vi "Post Build Script (G-CLI build).vi"(5 "create 7zip.bat only [T]":bool=TRUE, 6 "Package LabVIEW Version (19.0 (32-bit))":string, 7 "Project File Path":path, 8 "Package Source Folder":path, 9 "Package Version (major.minor.patch.build)":string, 10 "Product Name":string, 11 "Output Package File Path":path) -> (0 "error out":errorcluster)   [LabVIEW 2019, in "PostBuildSupport.lvclass"]
doc: "After you manually build the Application and Installer inside your project, you can then call this VI to create single self-extracting installer file. It is meant to be placed inside \"Post-Build Custom Action.vi\" that is called post VIPM package build."
uses:
  PostBuildSupport.lvclass
  PostBuildSupport.lvclass/PostBuildSupport.ctl
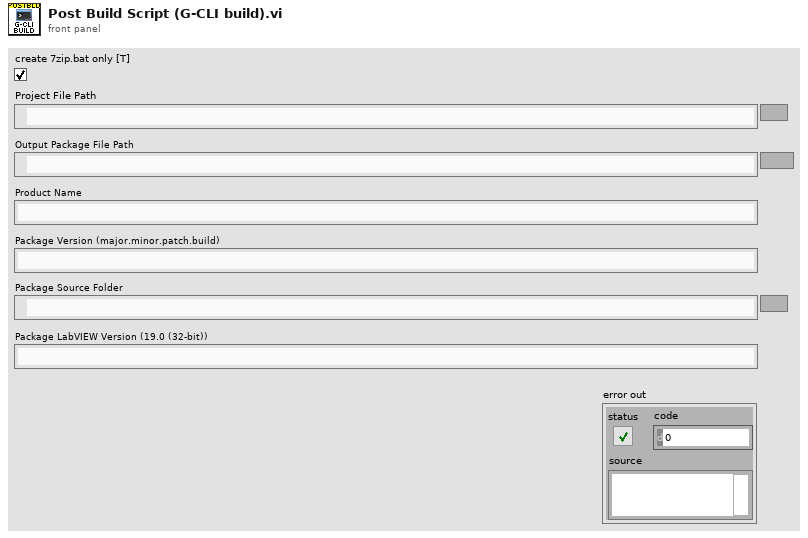
[diagram p1: front panel]
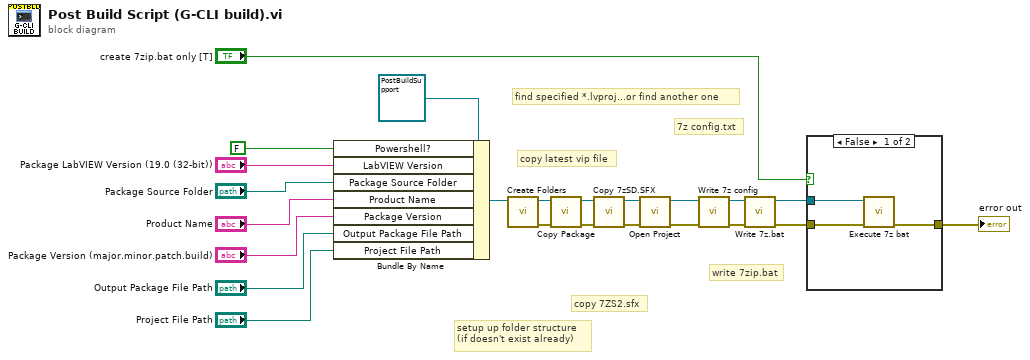
[diagram p0: block diagram]
diagram:
  # "find specified *.lvproj...or find another one"
  # "copy 7ZS2.sfx"
  # "setup up folder structure \n(if doesn't exist already)"
  # "copy latest vip file"
  # "7z config.txt"
  # "write 7zip.bat"
  n1 = Bundle By Name(cluster=refnum<class "PostBuildSupport.lvclass"> refnum ("PostBuildSupport in"), "Powershell?"=FALSE, "LabVIEW Version"="Package LabVIEW Version (19.0 (32-bit))", "Package Source Folder"="Package Source Folder", "Product Name"="Product Name", "Package Version"="Package Version (major.minor.patch.build)", "Output Package File Path"="Output Package File Path", "Project File Path"="Project File Path") -> (w18:refnum<class "PostBuildSupport.lvclass">)
  n2 = call "Create Folders.vi"("PostBuildSupport in"=w18) -> ("error out"=w17:errorcluster, "PostBuildSupport out"=w20:refnum<class "PostBuildSupport.lvclass">)  [unwired: 9 in]
  n3 = call "Copy Package.vi"("error in (no error)"=w17, "PostBuildSupport in"=w20) -> ("error out"=w16:errorcluster, "PostBuildSupport out"=w19:refnum<class "PostBuildSupport.lvclass">)  [unwired: 8 in]
  n4 = call "Copy 7zSD.SFX.vi"("error in (no error)"=w16, "PostBuildSupport in"=w19) -> ("error out"=w9:errorcluster, "PostBuildSupport out"=w8:refnum<class "PostBuildSupport.lvclass">)  [unwired: 8 in]
  n5 = call "Open Project.vi"("error in (no error)"=w9, "PostBuildSupport in"=w8) -> ("error out"=w6:errorcluster, "PostBuildSupport out"=w5:refnum<class "PostBuildSupport.lvclass">)  [unwired: 8 in]
  n6 = call "Write 7z config.vi"("error in (no error)"=w6, "PostBuildSupport in"=w5) -> ("error out"=w22:errorcluster, "PostBuildSupport out"=w23:refnum<class "PostBuildSupport.lvclass">)  [unwired: 8 in]
  n7 = call "Write 7z.bat.vi"("error in (no error)"=w22, "PostBuildSupport in"=w23) -> ("error out"=w11:errorcluster, "PostBuildSupport out"=w12:refnum<class "PostBuildSupport.lvclass">)  [unwired: 8 in]
  n8 = case shown="False" "create 7zip.bat only [T]" {
    tunnel: w12 -> [w26 _]
    tunnel: w11 -> [w25 w27]
    tunnel: [w24 w27] -> w10
    frame False {
      n9 = call "Execute 7z bat.vi"("error in (no error)"=w25, "PostBuildSupport in"=w26) -> ("error out"=w24:errorcluster)  [unwired: 8 in, 1 out]
    }
    frame True {
    }
  }
  "error out" <- w10
